vi "RendezvousRef.vi"(11 "Rendezvous Refnum":T1) -> (2 "Display string":string, 3 "Stop?":bool)   [LabVIEW 2017]
doc: "Displays the rendezvous name and size, the number of VIs or functions waiting to acquire the rendezvous, and the hex value of the reference. You can use this probe to set a breakpoint if the value is an invalid refnum."
uses:
  <vilib>/Utility/error.llb/DialogTypeEnum.ctl
panel:
  in  "error source":string="Rendezvous Refnum Probe"
  in  "Size":string="Size"
  in  "number waiting":string="Number waiting"
  in  "rendezvous name":string="Rendezvous name"
  in  "Pause if Not a Refnum":bool
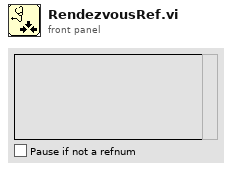
[diagram p1: front panel]
types:
  T1 = typedef "Rendezvous RefNum" = refnum<k1>
  T2 = typedef "DialogTypeEnum.ctl" = enum16{"no dialog", "OK message", "continue or stop message", "auto error handling dialog", "OK message + warnings", "continue/stop + warnings"}
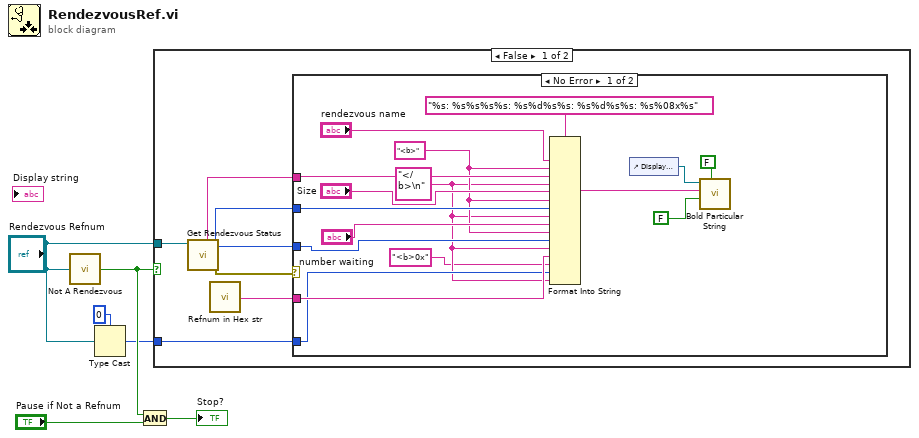
[diagram p0: block diagram]
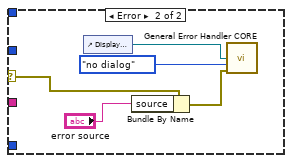
[diagram p2: hidden frame]
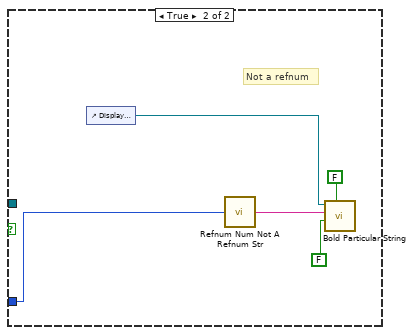
[diagram p3: hidden frame]
diagram:
  n1 = call <vilib>:"Not A Rendezvous.vi"("rendezvous"="Rendezvous Refnum") -> ("not a rendezvous"=w6:bool)
  n2 = Type Cast(type=u32 0, x="Rendezvous Refnum") -> (*(type *) &x=w1:u32)
  n3 = And(x=w6, y="Pause if Not a Refnum") -> (x .and. y?=→"Stop?":bool)
  n4 = case shown="False" w6 {
    tunnel: "Rendezvous Refnum" -> [w12 _]
    tunnel: w1 -> [w8 w36]
    frame False {
      n5 = call <vilib>:"Get Rendezvous Status.vi"("rendezvous"=w12) -> ("error out"=w13:errorcluster, "size"=w11:i32, "# waiting"=w10:i32, "name"=w9:string)  [unwired: 6 in, 1 out]
      n6 = call <vilib>:"Refnum in Hex str.vi"() -> ("refnum in hex"=w7:string)
      n7 = case shown="No Error" w13 {
        selector: w13 -> [_ w32]
        tunnel: w8 -> [w17 _]
        tunnel: w11 -> [w22 _]
        tunnel: w9 -> [w24 _]
        tunnel: w10 -> [w20 _]
        tunnel: w7 -> [w19 _]
        frame No Error {
          w16 = "</b>\n"
          w18 = "<b>"
          n8 = Format Into String(format string="%s: %s%s%s%s: %s%d%s%s: %s%d%s%s: %s%08x%s", "rendezvous name", w18, w24, w16, "Size", w18, w22, w16, "number waiting", w18, w20, w16, w19, "<b>0x", w17, w16) -> (resulting string=w28:string)  [unwired: 2 in, 1 out]
          n9 = control-ref of="Display string"() -> (w29:refnum<vi>)
          n10 = call <vilib>:"Bold Particular String.vi"("Always Refresh? (TRUE)"=FALSE ("Always Refresh? (FALSE)"), "resize string? (TRUE)"=FALSE ("resize string?"), "text to display"=w28, "string refnum"=w29) -> ()  [unwired: 6 in, 2 out]
        }
        frame Error {
          n11 = control-ref of="Display string"() -> (w31:refnum<vi>)
          n12 = Bundle By Name(cluster=w32, "source"="error source") -> (w33:errorcluster)
          n13 = call <vilib>:"General Error Handler CORE.vi"("String to Format (not a refnum)"=w31, "type of dialog (OK msg:1)"=DialogTypeEnum."no dialog", "error in (no error)"=w33) -> ()  [unwired: 7 in, 6 out]
        }
      }
    }
    frame True {
      # "Not a refnum"
      n14 = control-ref of="Display string"() -> (w38:refnum<vi>)
      n15 = call <vilib>:"Refnum Num Not A Refnum Str.vi"("Numeric"=w36) -> ("text to display"=w35:string)
      n16 = call <vilib>:"Bold Particular String.vi"("Always Refresh? (TRUE)"=FALSE ("Always Refresh? (FALSE)"), "resize string? (TRUE)"=FALSE, "text to display"=w35, "string refnum"=w38) -> ()  [unwired: 6 in, 2 out]
    }
  }
